vi "Destroy.vi"(8 "Error In":errorcluster, 11 "WebView in":refnum<class "WebView.lvclass">) -> (0 "Error Out":errorcluster)   [LabVIEW 2024, in "WebView.lvclass"]
uses:
  WebView.lvclass
  WebView.lvclass/WebView.ctl
  <vilib>/sklein/WebView2/Libs/Microsoft.Web.WebView2.Core.dll
  <vilib>/sklein/WebView2/Libs/Microsoft.Web.WebView2.WinForms.dll
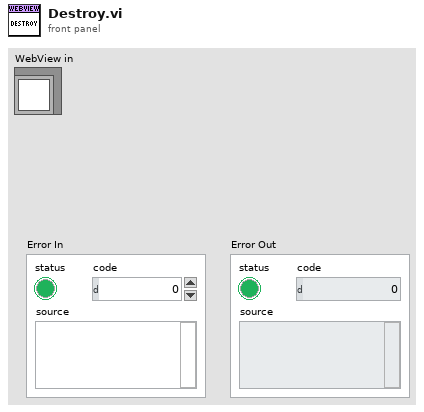
[diagram p1: front panel]
types:
  T1 = typedef "WebView.lvclass/Resources--cluster.ctl" = cluster{"WebView2 Control":refnum<k24>, "Webview2 Core":refnum<k24>, "event callback":refnum<k27>, "Environment":refnum<k24>}
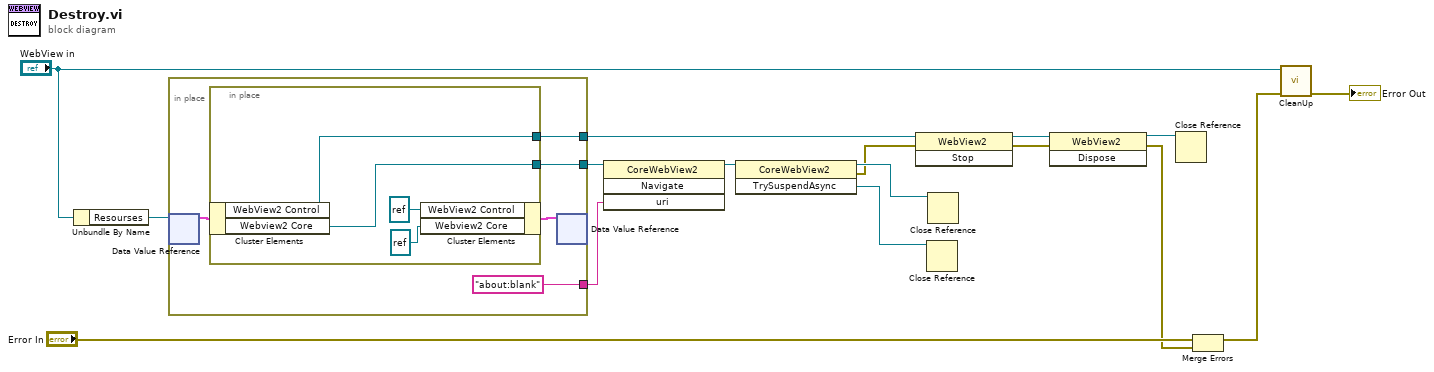
[diagram p0: block diagram]
diagram:
  n1 = Unbundle By Name("WebView in") -> ("Resourses"=w12:refnum<data-value>)
  n2 = in-place {
    in-place-border: ["about:blank" ("uri")] -> w14
    in-place-border: [w20] -> w13
    in-place-border: [w17] -> w11
    n3 = in-place-dvr #1(w12) -> (w19:T1)  [unwired: 1 out]
    n4 = in-place {
      in-place-border: [w25] -> w20
      in-place-border: [w23] -> w17
      n5 = in-place-cluster #2(w19) -> ("WebView2 Control"=w23:refnum<k24>, "Webview2 Core"=w25:refnum<k24>)
      n6 = in-place-cluster #2("WebView2 Control"=refnum<k24> refnum ("WebView2"), "Webview2 Core"=refnum<k24> refnum) -> (w18:T1)
    }
    n7 = in-place-dvr #1(w18) -> ()  [unwired: 2 out]
  }
  n8 = invoke class="CoreWebView2" method="Navigate"(reference=w13, "uri"=w14) -> (reference out=w15:refnum<k24>)  [unwired: 2 in, 3 out]
  n9 = invoke class="CoreWebView2" method="TrySuspendAsync"(reference=w15) -> (reference out=w7:refnum<k24>, error out=w6:errorcluster, "TrySuspendAsync"=w8:refnum<k24>)  [unwired: 2 in]
  n10 = invoke class="WebView2" method="Stop"(reference=w11, error in=w6) -> (reference out=w10:refnum<k24>, error out=w9:errorcluster)  [unwired: 1 in, 1 out]
  n11 = Close Reference(reference=w8) -> ()  [unwired: 1 in, 1 out]
  n12 = Close Reference(reference=w7) -> ()  [unwired: 1 in, 1 out]
  n13 = invoke class="WebView2" method="Dispose"(reference=w10, error in=w9) -> (reference out=w5:refnum<k24>, error out=w4:errorcluster)  [unwired: 1 in, 1 out]
  n14 = Close Reference(reference=w5) -> ()  [unwired: 1 in, 1 out]
  n15 = Merge Errors("Error In", w4) -> (w2:errorcluster)
  n16 = call "CleanUp.vi"("Error In"=w2, "WebView in"="WebView in") -> ("Error Out"=→"Error Out":errorcluster)  [unwired: 9 in]
